vi "VI Server_Defer FP Update_CheckStatus.vi"(8 "error in":errorcluster, 11 "VI Server Cluster":T1={"Labels"=["Label", "Size", "Font", "Heght", "Width", "Ledding Denominator", "Ledding Nominator", "Label Number", "Microstep Resolution", "X", "Y", "Z", "Italic?", "Underlined?"], "Refs"=[], "VI Ref"=refnum}) -> (0 "error out":errorcluster, 2 "Defer Panel Updates.Status":bool, 3 "VI Server Cluster.DUP":T1={"Labels"=["Label", "Size", "Font", "Heght", "Width", "Ledding Denominator", "Ledding Nominator", "Label Number", "Microstep Resolution", "X", "Y", "Z", "Italic?", "Underlined?"], "Refs"=[], "VI Ref"=refnum})   [LabVIEW 2020, in "VI Server Toolkit LV2013.lvlib"]
doc: "Checks if the Front Panel update is being deferred.\nThis VI is helpful for debugging purposes when multiple FP updates are managed and may conflict with each other."
uses:
  VI Server Toolkit LV2013.lvlib
  VI Server_TypeDefs/VI Server_RefsCluster.ctl
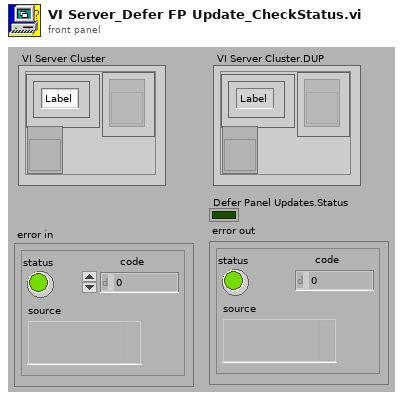
[diagram p1: front panel]
types:
  T1 = typedef "VI Server_RefsCluster.ctl" = cluster{"Labels":string[], "Refs":refnum<vi>[], "VI Ref":refnum<vi>}
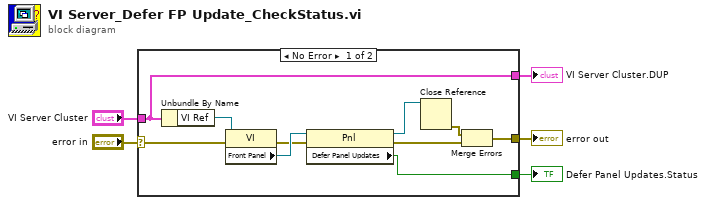
[diagram p0: block diagram]
diagram:
  n1 = case shown="No Error" "error in" {
    selector: "error in" -> [w7 w17]
    tunnel: "VI Server Cluster" -> [w6 w16]
    tunnel: [w12 _] -> w2
    tunnel: [w8 w17] -> w3
    tunnel: [w6 w16] -> w5
    frame No Error {
      n2 = Unbundle By Name(w6) -> ("VI Ref"=w15:refnum<vi>)
      n3 = property class="VI"(reference=w15, error in=w7) -> (error out=w13:errorcluster, "Front Panel"=w14:refnum<vi>)  [unwired: 1 out]
      n4 = property class="Pnl"(reference=w14, error in=w13) -> (reference out=w9:refnum<vi>, error out=w11:errorcluster, "Defer Panel Updates"=w12:bool)
      n5 = Close Reference(reference=w9) -> (error out=w10:errorcluster)  [unwired: 1 in]
      n6 = Merge Errors(w10, w11) -> (w8:errorcluster)
    }
    frame Error {
    }
  }
  "VI Server Cluster.DUP" <- w5
  "error out" <- w3
  "Defer Panel Updates.Status" <- w2
